vi "Initialize.vi"(8 "error in (no error)":errorcluster, 11 "PXI_MultiTrig in":refnum<class "PXI_MultiTrig.lvclass">) -> (0 "error out":errorcluster, 3 "PXI_MultiTrig out":refnum<class "PXI_MultiTrig.lvclass">)   [LabVIEW 2014, in "SyncPlugins.lvlib" / "PXI_MultiTrig.lvclass"]
uses:
  PXI_MultiTrig.lvclass
  PXI_MultiTrig.lvclass/PXI_MultiTrig.ctl
  Accessors/Read Clocks.vi
  Accessors/Read Triggers.vi
  Accessors/Write SysHandle.vi
  Accessors/Write SysRef.vi
  Accessors/Read SyncWindowsClock.vi
  <vilib>/Utility/error.llb/Error Cluster From Error Code.vi
  <vilib>/ErrorRing/Error Ring.xnode
  <vilib>/nisyscfg/nisyscfg.lvlib
  <resource>/objmgr/niflexriosae.rc
  <resource>/objmgr/nisysapi.rc
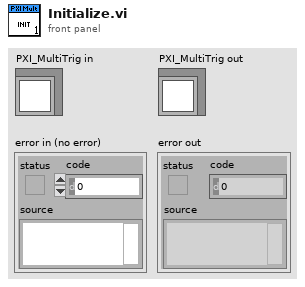
[diagram p1: front panel]
types:
  T1 = typedef "SyncPlugins.lvlib/PXI_MultiTrig.lvclass/clClocks.ctl" = cluster{"Name":string, "RefClk":string, "ClkTerminal":string, "Frequency":dbl, "DutyCycle":dbl, "ClkType":string, "Initiated":bool, "TrigTime":bool}
  T2 = typedef "SyncPlugins.lvlib/PXI_MultiTrig.lvclass/clTrigger.ctl" = cluster{"Name":string, "DestTerm":string, "SrcTerm":string, "SyncClk":string, "Edge":i32, "Invert?":i32, "Initiated":bool, "Type":string, "TrigTime":bool}
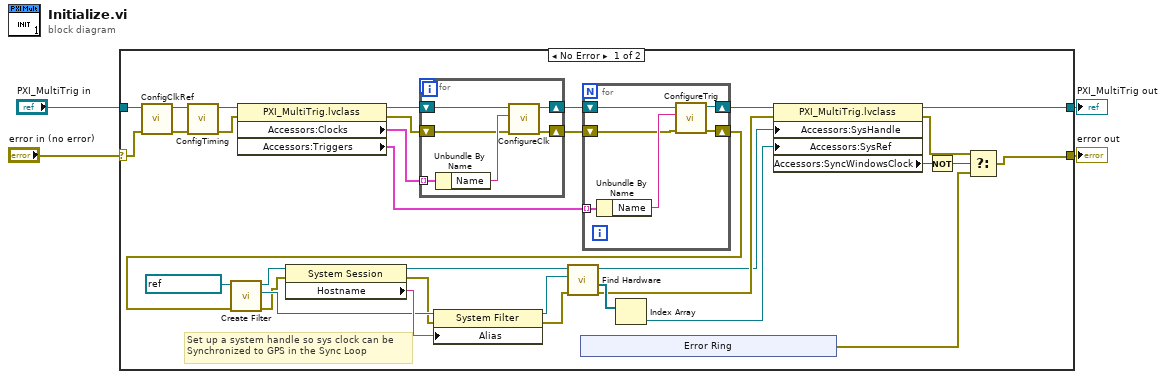
[diagram p0: block diagram]
diagram:
  n1 = case shown="No Error" "error in (no error)" {
    selector: "error in (no error)" -> [w31 w55]
    tunnel: "PXI_MultiTrig in" -> [w32 w56]
    tunnel: [w13 w56] -> w2
    tunnel: [w5 w55] -> w1
    frame No Error {
      # "Set up a system handle so sys clock can be\nSynchronized to GPS in the Sync Loop"
      n2 = call "ConfigClkRef.vi"("error in (no error)"=w31, "PXI_MultiTrig in"=w32) -> ("error out"=w29:errorcluster, "PXI_MultiTrig out"=w30:refnum<class "PXI_MultiTrig.lvclass">)  [unwired: 8 in]
      n3 = call "ConfigTiming.vi"("error in (no error)"=w29, "PXI_MultiTrig in"=w30) -> ("error out"=w27:errorcluster, "PXI_MultiTrig out"=w28:refnum<class "PXI_MultiTrig.lvclass">)  [unwired: 8 in]
      n4 = property class="PXI_MultiTrig.lvclass"(reference=w28, error in=w27) -> (reference out=w37:refnum<class "PXI_MultiTrig.lvclass">, error out=w36:errorcluster, "Accessors:Clocks"=w26:T1[], "Accessors:Triggers"=w25:T2[])
      n5 = for {
        tunnel: w26 -> [w54] mode=indexing
        shift-right: [w50] -> w35
        shift-left: w37 -> [w53]
        shift-right: [w49] -> w34
        shift-left: w36 -> [w51]
        n6 = Unbundle By Name(w54) -> ("Name"=w52:string)
        n7 = call-dynamic "ConfigureClk.vi"("error in (no error)"=w51, "ClkName"=w52, "PXI_MultiTrig in"=w53) -> ("error out"=w49:errorcluster, "PXI_MultiTrig out"=w50:refnum<class "PXI_MultiTrig.lvclass">)  [unwired: 7 in]
      }
      n8 = xnode "Error Ring"() -> ("error out"=w6:errorcluster)
      n9 = for {
        shift-right: [w44] -> w33
        shift-left: w35 -> [w43]
        tunnel: w25 -> [w48] mode=indexing
        shift-right: [w45] -> w16
        shift-left: w34 -> [w46]
        n10 = Unbundle By Name(w48) -> ("Name"=w47:string)
        n11 = call-dynamic "ConfigureTrig.vi"("error in (no error)"=w46, "TrigName"=w47, "PXI_MultiTrig in"=w43) -> ("error out"=w45:errorcluster, "PXI_MultiTrig out"=w44:refnum<class "PXI_MultiTrig.lvclass">)  [unwired: 7 in]
      }
      n12 = call <vilib>:"Create Filter.vi"("error in (no error)"=w16, "Session in"=refnum<k21> "localhost") -> ("error out"=w15:errorcluster, "Filter out"=w17:refnum<k20>, "Session out"=w19:refnum<k21>)  [unwired: 7 in]
      n13 = property class="System Session"(reference=w19, error in=w15) -> (reference out=w21:refnum<k21>, error out=w14:errorcluster, "Hostname"=w20:string)
      n14 = property class="System Filter"(reference=w17, error in=w14, "Alias"=w20) -> (reference out=w22:refnum<k20>, error out=w23:errorcluster)
      n15 = call <vilib>:"Find Hardware.vi"("error in (no error)"=w23, "Filter in"=w22, "Session in"=w21) -> ("error out"=w12:errorcluster, "Resources out"=w24:refnum<k20>[], "Session out"=w11:refnum<k21>)  [unwired: 5 in, 1 out]
      n16 = Index Array(array=w24) -> (element=w10:refnum<k20>)  [unwired: 1 in]
      n17 = property class="PXI_MultiTrig.lvclass"(reference=w33, error in=w12, "Accessors:SysHandle"=w11, "Accessors:SysRef"=w10) -> (reference out=w13:refnum<class "PXI_MultiTrig.lvclass">, error out=w9:errorcluster, "Accessors:SyncWindowsClock"=w8:bool)
      n18 = Not(x=w8) -> (.not. x?=w7:bool)
      n19 = Select(t=w9, s=w7, f=w6) -> (s? t:f=w5:errorcluster)
    }
    frame Error {
    }
  }
  "error out" <- w1
  "PXI_MultiTrig out" <- w2
